vi "Get Data Type.vi"(1 "Data Type Index":u16) -> (0 "Data Type Name":string)   [LabVIEW 2020]
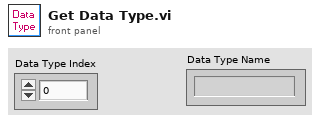
[diagram p1: front panel]
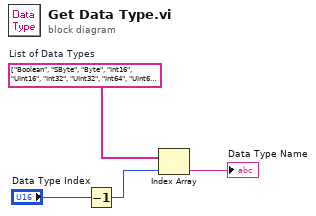
[diagram p0: block diagram]
diagram:
  w4 = string[] ["Boolean", "SByte", "Byte", "Int16", "UInt16", "Int32", "UInt32", "Int64", "UInt64", "Float", "Double", "String", "DateTime", "ByteString", "Array of Boolean", "Array of SByte", "Array of Byte", "Array of Int16", "Array of UInt16", "Array of Int32", "Array of UInt32", "Array of Int64", "Array of UInt64", "Array of Float", "Array of Double", "Array of String", "Array of DateTime", "Array of ByteString"]  # List of Data Types
  n1 = Decrement(x="Data Type Index") -> (x-1=w1:u16)
  n2 = Index Array(array=w4, index=w1) -> (element=→"Data Type Name":string)
